vi "Test Create Logger with File Sink as Default Config.vi"(11 "Test Case In":refnum<class "File Sink.lvclass">) -> (0 "error out":errorcluster, 3 "Test Case Out":refnum<class "File Sink.lvclass">)   [LabVIEW 2020, in "File Sink.lvclass"]
uses:
  File Sink.lvclass
  C:/Program Files (x86)/National Instruments/LabVIEW 2020/vi.lib/Astemes/LUnit/Test Case.lvclass
  Source/Type Defs/Debug Level.ctl
  <vilib>/Astemes/LUnit/Test Case.lvclass/Test Case.ctl
  e94ff1bf-c1b1-42c1-a6e3-1538fdc900a3.vi
  4993e8ee-a06a-463a-9684-69129f64d5ce.vi
  ebeb964f-1c40-45c4-b7ad-328f89dac856.vi
  <vilib>/Astemes/LUnit/Core/LUnit Test Case/Private/Append Fail Result.vi
  <vilib>/Astemes/LUnit/Core/LUnit Test Case/Private/Append Pass Result.vi
  e94ff1bf-c1b1-42c1-a6e3-1538fdc900a3.vi/9c5d11cd-9439-4240-a1ee-d9baace9c924.vi
  4993e8ee-a06a-463a-9684-69129f64d5ce.vi/9c5d11cd-9439-4240-a1ee-d9baace9c924.vi
  ebeb964f-1c40-45c4-b7ad-328f89dac856.vi/9c5d11cd-9439-4240-a1ee-d9baace9c924.vi
  <vilib>/Astemes/LUnit/Core/LUnit Test Case/Private/Run In UI.vi
  <vilib>/Utility/error.llb/Clear Errors.vi
  Source/Sinks/File Sink/File Sink.lvclass
  C:/Users/hughe_cx/Documents/05_repos/LVLog/Source/Sinks/Sink/Sink.lvclass
  <vilib>/Astemes/LUnit/Test Case.lvclass
  Source/LV Log.lvlib
  Source/Logger/Logger.lvclass
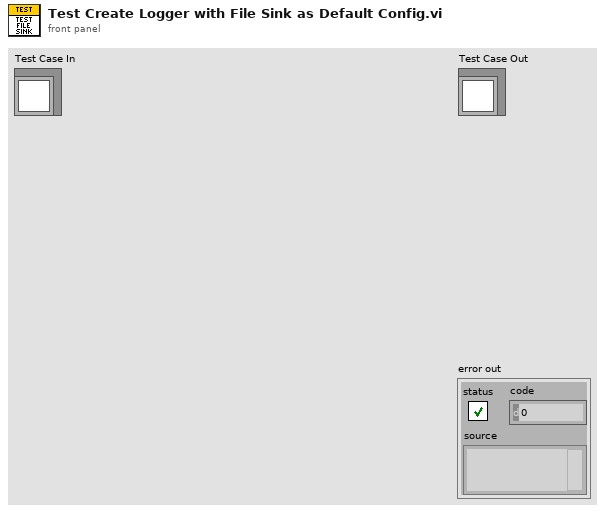
[diagram p1: front panel]
types:
  T1 = typedef "LV Log.lvlib/Debug Level.ctl" = enum16{"DEFAULT", "DEBUG", "INFO", "WARN", "ERROR", "FATAL"}
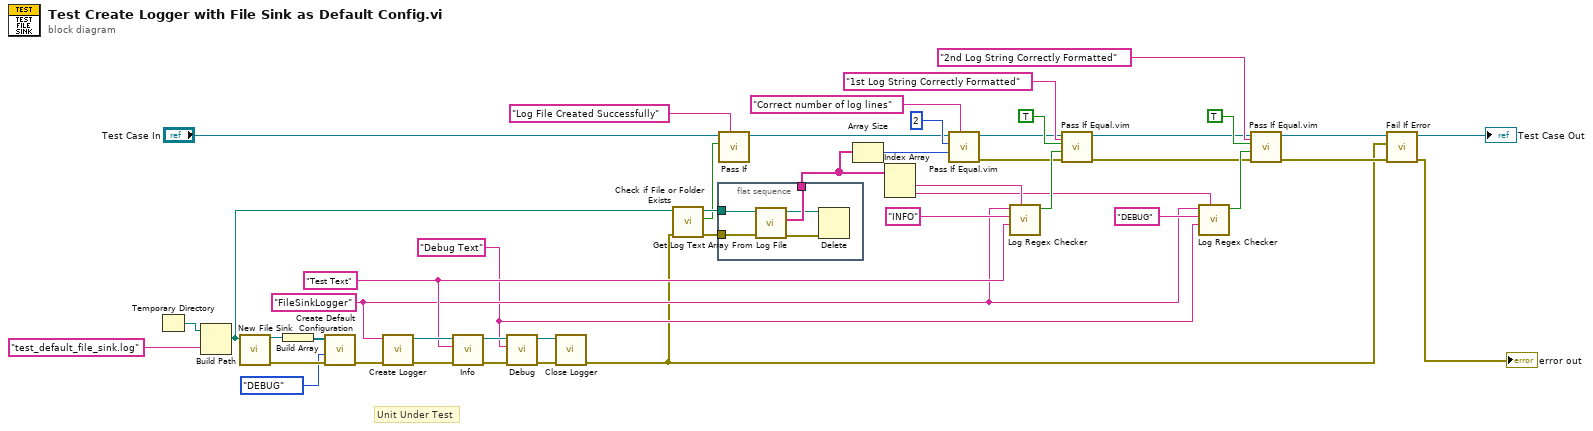
[diagram p0: block diagram]
diagram:
  w25 = "Debug Text" ("Log Text")
  w35 = "Test Text" ("Log Text")
  w26 = "FileSinkLogger" ("Name")
  # "Unit Under Test"
  n1 = Temporary Directory() -> (w41:path)
  n2 = Build Path(base path=w41, name or relative path="test_default_file_sink.log" ("format string")) -> (appended path=w10:path)
  n3 = call "New File Sink.vi"("File Path"=w10) -> ("error out"=w43:errorcluster, "File Sink out"=w12:refnum<class "File Sink.lvclass">)  [unwired: 9 in]
  n4 = Build Array(w12) -> (w42:refnum<class "File Sink.lvclass">[])
  n5 = call "Create Default Configuration.vi"("Sinks"=w42, "Debug Level in"=Debug_Level."DEBUG", "error in (no error)"=w43) -> ("error out"=w44:errorcluster)  [unwired: 7 in]
  n6 = call "Create Logger.vi"("error in (no error)"=w44, "Name"=w26) -> ("error out"=w39:errorcluster, "Logger out"=w38:refnum<class "Logger.lvclass">)  [unwired: 8 in]
  n7 = call "Info.vi"("error in (no error)"=w39, "Log Text"=w35, "Logger in"=w38) -> ("error out"=w34:errorcluster, "Logger out"=w33:refnum<class "Logger.lvclass">)  [unwired: 6 in, 1 out]
  n8 = call "Debug.vi"("error in (no error)"=w34, "Log Text"=w25, "Logger in"=w33) -> ("error out"=w4:errorcluster, "Logger out"=w3:refnum<class "Logger.lvclass">)  [unwired: 6 in, 1 out]
  n9 = call "Close Logger.vi"("error in (no error)"=w4, "Logger in"=w3) -> ("error out"=w2:errorcluster)  [unwired: 9 in]
  n10 = call <vilib>:"Check if File or Folder Exists.vi"("error in (no error)"=w2, "path"=w10) -> ("error out"=w9:errorcluster, "file or folder exists?"=w6:bool, "dup path"=w11:path)  [unwired: 7 in]
  n11 = flat-sequence {
    tunnel: w11 -> [w51]
    tunnel: [w50] -> w19
    tunnel: w9 -> [w47]
    frame #0 {
      n12 = call "Get Log Text Array From Log File.vi"("error in"=w47, "Log File Path in"=w51) -> ("error out"=w49:errorcluster, "Log Text Array"=w50:string[], "Log File Path out"=w48:path)  [unwired: 7 in]
      n13 = Delete(path (use dialog)=w48, error in=w49) -> ()  [unwired: 3 in, 3 out]
    }
  }
  n14 = call <vilib>:"Pass If.vi"("Description"="Log File Created Successfully", "Pass?"=w6, "LUnit Test Case In"="Test Case In") -> ("LUnit Test Case Out"=w7:refnum<class "File Sink.lvclass">)  [unwired: 7 in, 1 out]
  n15 = Array Size(array=w19) -> (size(s)=w18:i32)
  n16 = Index Array(array=w19) -> (element #1=w24:string, element #2=w23:string)  [unwired: 2 in]
  n17 = call "Pass If Equal.vim"("Description"="Correct number of log lines", "Actual"=w18, "Expected"=2, "LUnit Test Case In"=w7) -> ("error out"=w13:errorcluster, "LUnit Test Case Out"=w20:refnum<class "File Sink.lvclass">)  [unwired: 6 in]
  n18 = call "Log Regex Checker.vi"("Log String"=w24, "Expected Log Text (Any)"=w35, "Expected Log Level (Any)"="INFO", "Expected Logger Name (Any)"=w26) -> ("Math Found"=w31:bool)  [unwired: 5 in, 2 out]
  n19 = call "Pass If Equal.vim"("Description"="1st Log String Correctly Formatted", "error in (no error)"=w13, "Actual"=w31, "Expected"=TRUE, "LUnit Test Case In"=w20) -> ("error out"=w14:errorcluster, "LUnit Test Case Out"=w22:refnum<class "File Sink.lvclass">)  [unwired: 5 in]
  n20 = call "Log Regex Checker.vi"("Log String"=w23, "Expected Log Text (Any)"=w25, "Expected Log Level (Any)"="DEBUG", "Expected Logger Name (Any)"=w26) -> ("Math Found"=w30:bool)  [unwired: 5 in, 2 out]
  n21 = call "Pass If Equal.vim"("Description"="2nd Log String Correctly Formatted", "error in (no error)"=w14, "Actual"=w30, "Expected"=TRUE, "LUnit Test Case In"=w22) -> ("error out"=w15:errorcluster, "LUnit Test Case Out"=w21:refnum<class "File Sink.lvclass">)  [unwired: 5 in]
  n22 = call <vilib>:"Fail If Error.vi"("error in (no error)"=w15, "Assert error"=w2, "LUnit Test Case In"=w21) -> ("error out"=→"error out":errorcluster, "LUnit Test Case Out"=→"Test Case Out":refnum<class "File Sink.lvclass">)  [unwired: 7 in]
